vi "Validate User Input.vi"(8 "error in (no error)":errorcluster, 9 "available measurements name":string[](array[string]), 10 "project ref":refnum<vi>, 11 "multicolumnListbox in":refnum<vi>) -> (0 "error out":errorcluster, 2 "warning?":bool, 3 "multicolumnListbox out":refnum<vi>)   [LabVIEW 2021, in "Create Measurement Plug-In Client.lvlib"]
uses:
  Create Measurement Plug-In Client.lvlib
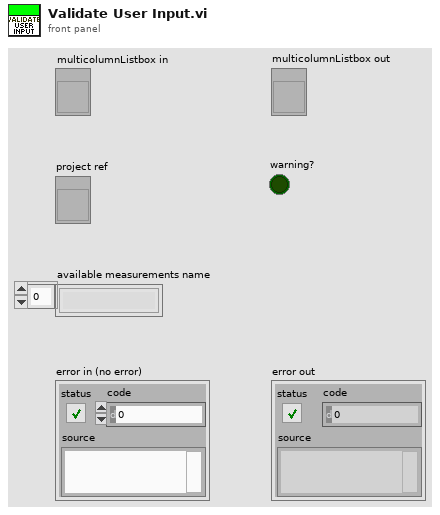
[diagram p1: front panel]
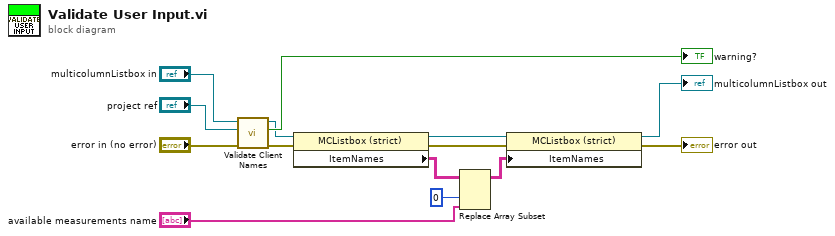
[diagram p0: block diagram]
diagram:
  n1 = call "Validate Client Names.vi"("error in (no error)"="error in (no error)", "project ref"="project ref", "multicolumnListbox in"="multicolumnListbox in") -> ("error out"=w12:errorcluster, "warning?"=→"warning?":bool, "multicolumnListbox out"=w8:refnum<vi>)  [unwired: 6 in]
  n2 = property class="MCListbox (strict)"(reference=w8, error in=w12) -> (reference out=w3:refnum<vi>, error out=w9:errorcluster, "ItemNames"=w7:string[][])
  n3 = Replace Array Subset(array=w7, new element="available measurements name", index (col)=0 ("disabled index (col)")) -> (w2:string[][])  [unwired: 1 in]
  n4 = property class="MCListbox (strict)"(reference=w3, error in=w9, "ItemNames"=w2) -> (reference out=→"multicolumnListbox out":refnum<vi>, error out=→"error out":errorcluster)
